vi "Ait 664 - Add Input VLs.vi"(0 "Item Ref in":T1 format="%.0x", 5 "Input VL":T2, 11 "error in (no error)":errorcluster) -> (4 "Item Ref out":T1 format="%.0x", 15 "error out":errorcluster)   [LabVIEW 2013, in "AIT 664 Custom Device.lvlib"]
doc: "Populate Input VL Page"
uses:
  AIT 664 Custom Device.lvlib
  Controls/664 - XML Input VL.ctl
  Controls/664 - XML Rx Message Port.ctl
  Controls/664 - Sampling Type.ctl
  Controls/664 -Param.ctl
  <vilib>/NI Veristand/Custom Device API/Custom Device Item Ref.ctl
  Controls and Global/Global.vi
  <vilib>/NI Veristand/Custom Device API/Set Item Property (U32).vi
  <vilib>/NI Veristand/Custom Device API/Custom Device API.lvlib
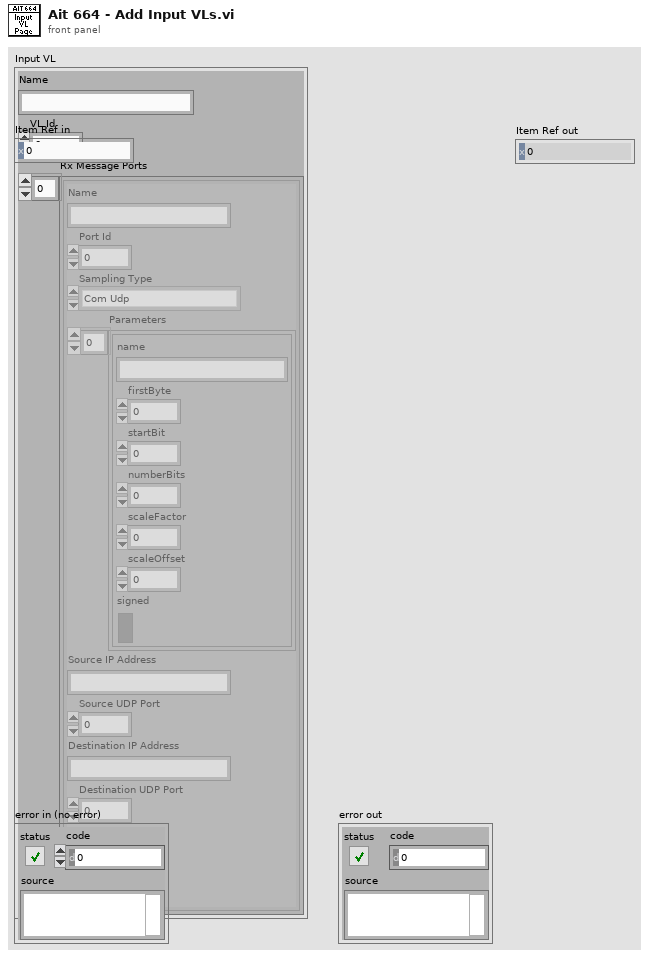
[diagram p1: front panel]
types:
  T1 = typedef "Custom Device API.lvlib/Custom Device Item Ref.ctl" = u64
  T2 = typedef "AIT 664 Custom Device.lvlib/664 - XML Input VL.ctl" = cluster{"Name":string, "VL Id":u32, "Rx Message Ports":T3[]}
  T3 = typedef "AIT 664 Custom Device.lvlib/664 - XML Rx Message Port.ctl" = cluster{"Name":string, "Port Id":u32, "Sampling Type":T4, "Parameters":T5[], "Source IP Address":string, "Source UDP Port":u32, "Destination IP Address":string, "Destination UDP Port":u32, "Rx Rate (ms)":u32, "Buffer Depth":u32}
  T4 = typedef "AIT 664 Custom Device.lvlib/664 - Sampling Type.ctl" = enum16{"Com Udp", "Com Udp Queuing", "Sap Udp", "Sap Ip", "Sap Mac", "Unknown"}
  T5 = typedef "AIT 664 Custom Device.lvlib/664 -Param.ctl" = cluster{"name":string, "firstByte":i32, "startBit":i32, "numberBits":i32, "scaleFactor":dbl, "scaleOffset":dbl, "signed":bool}
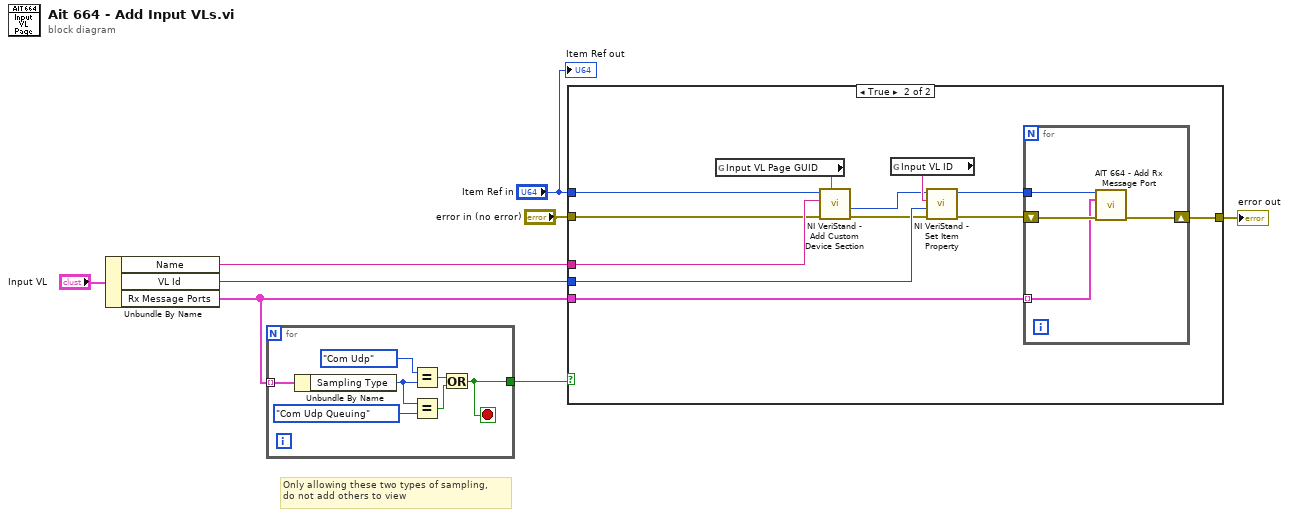
[diagram p0: block diagram]
diagram:
  # "Only allowing these two types of sampling,\ndo not add others to view"
  n1 = Unbundle By Name("Input VL") -> ("Name"=w7:string, "VL Id"=w8:u32, "Rx Message Ports"=w4:T3[])
  n2 = for {
    tunnel: w4 -> [w15] mode=indexing
    tunnel: [w9] -> w3
    stop <- w9 stop-if-true
    n3 = Unbundle By Name(w15) -> ("Sampling Type"=w13:T4)
    n4 = Equal?(x=664_-_Sampling_Type."Com Udp" ("Sampling Type"), y=w13) -> (x = y?=w11:bool)
    n5 = Equal?(x=w13, y=664_-_Sampling_Type."Com Udp Queuing" ("Sampling Type")) -> (x = y?=w10:bool)
    n6 = Or(x=w11, y=w10) -> (x .or. y?=w9:bool)
  }
  n7 = case shown="True" w3 {
    tunnel: w8 -> [_ w27]
    tunnel: w7 -> [_ w24]
    tunnel: w4 -> [_ w22]
    tunnel: [w16 w19] -> w5
    tunnel: "error in (no error)" -> [w16 w18]
    tunnel: "Item Ref in" -> [_ w17]
    frame False {
    }
    frame True {
      n8 = global read "Global.vi" "Input VL Page GUID"() -> (w23:string)
      n9 = call <vilib>:"NI VeriStand - Add Custom Device Section.vi"("GUID (Default Section)"=w23, "error in (no error)"=w18, "Section Name"=w24, "Parent Ref in"=w17) -> ("error out"=w25:errorcluster, "Section Ptr"=w26:T1)  [unwired: 4 in, 2 out]
      n10 = global read "Global.vi" "Input VL ID"() -> (w28:string)
      n11 = call-poly <vilib>:"NI VeriStand - Set Item Property.vi"("error in (no error)"=w25, "Value"=w27, "Property Name"=w28, "Item Ref in"=w26) -> ("error out"=w21:errorcluster, "Item Ref out"=w20:T1)  [unwired: 5 in, 1 out]
      n12 = for {
        tunnel: w22 -> [w31] mode=indexing
        tunnel: w20 -> [w30]
        shift-right: [w29] -> w19
        shift-left: w21 -> [w32]
        n13 = call "AIT 664 - Add Rx Message Port.vi"("Item Ref in"=w30, "Rx Message Port"=w31, "error in (no error)"=w32) -> ("error out"=w29:errorcluster)  [unwired: 12 in]
      }
    }
  }
  "error out" <- w5
  "Item Ref out" <- "Item Ref in"
